vi "Write.vi"(8 "error in (no error)":errorcluster, 10 "Byte Array":u8[](array[numeric]), 11 "VISA resource name":refnum<visa-resource-name>) -> (0 "error out":errorcluster, 3 "VISA resource name out":refnum<visa-resource-name>)   [LabVIEW 2009, in "Digikrom DK24x.lvlib"]
doc: "Writes the data in \"string to write\" to the VISA resource."
uses:
  Digikrom DK24x.lvlib
panel:
  out "string to write":string
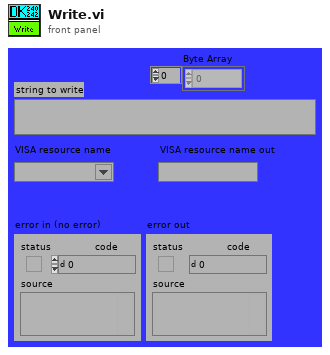
[diagram p1: front panel]
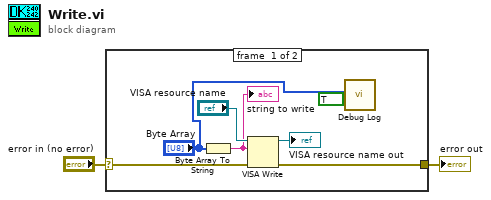
[diagram p0: block diagram]
diagram:
  n1 = case shown="No Error" "error in (no error)" {
    selector: "error in (no error)" -> [w6 w10]
    tunnel: [w7 w10] -> w1
    frame #0 {
      n2 = Byte Array To String(unsigned byte array="Byte Array") -> (string=w5:string)
      "string to write" <- w5
      n3 = VISA Write(VISA resource name="VISA resource name", write buffer=w5, error in (no error)=w6) -> (VISA resource name out=→"VISA resource name out":refnum<visa-resource-name>, error out=w7:errorcluster)  [unwired: 1 out]
      n4 = call "Debug Log.vi"("Write?"=TRUE, "Data"="Byte Array") -> ()  [unwired: 1 in, 9 out]
    }
    frame #1 {
    }
  }
  "error out" <- w1
